vi "Open.vi"(8 "error in":errorcluster, 9 "parameters":variant, 10 "file path":path, 11 "repository in":refnum<class "NISE_CEF_Repository.lvclass">) -> (0 "error out":errorcluster, 2 "invalid?":bool, 3 "repository out":refnum<class "NISE_CEF_Repository.lvclass">)   [LabVIEW 2013, in "NISE_CEF_Repository.lvclass"]
doc: "Loads the saved information of the repo. It could load multiple files at the same time. An option to add file versioning could be included in the files, and the code to manage changes would be in this VI."
uses:
  NISE_CEF_Repository.lvclass
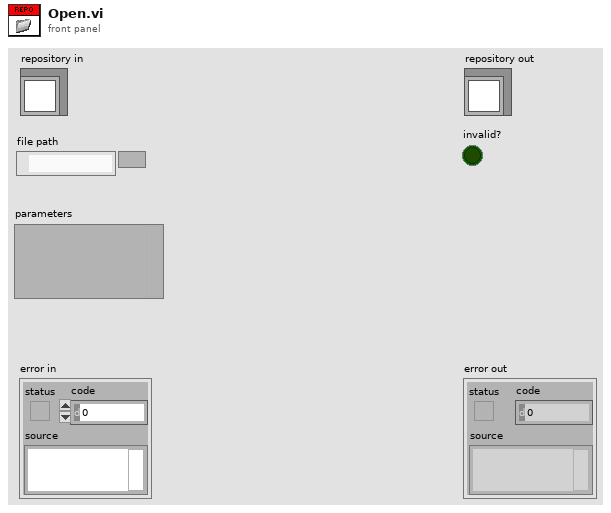
[diagram p1: front panel]
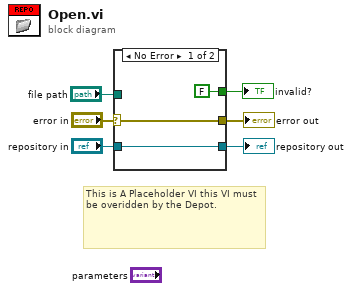
[diagram p0: block diagram]
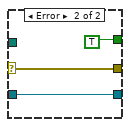
[diagram p2: hidden frame]
diagram:
  # "This is A Placeholder VI this VI must be overidden by the Depot."
  n1 = case shown="No Error" "error in" {
    selector: "error in" -> [w8 w12]
    tunnel: [w8 w12] -> w5
    tunnel: [w9 w11] -> w3
    tunnel: "repository in" -> [w9 w11]
    tunnel: "file path" -> [_ _]
    tunnel: [FALSE TRUE] -> w1
    frame No Error {
    }
    frame Error {
    }
  }
  "error out" <- w5
  "repository out" <- w3
  "invalid?" <- w1
